vi "UseOuterEnvelope.vi"(10 "Outer Envelope Label":string) -> (3 "Translator":refnum<class "AddOuterEnvelope.lvclass">)   [LabVIEW 2011, in "Messenging.lvlib" / "AddOuterEnvelope.lvclass"]
uses:
  AddOuterEnvelope.lvclass
  AddOuterEnvelope.lvclass/AddOuterEnvelope.ctl
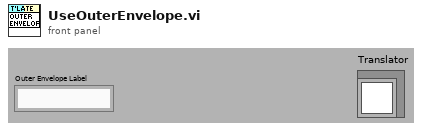
[diagram p1: front panel]
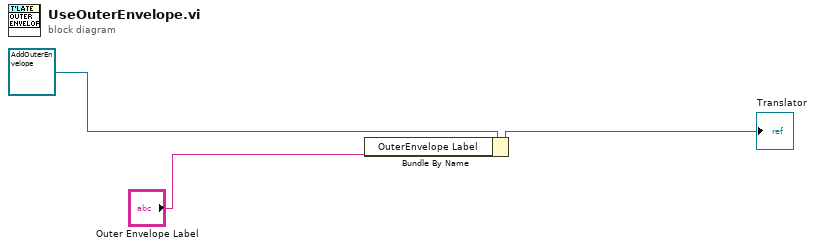
[diagram p0: block diagram]
diagram:
  n1 = Bundle By Name(cluster=refnum<class "AddOuterEnvelope.lvclass"> refnum ("SubstututeMessage in"), "OuterEnvelope Label"="Outer Envelope Label") -> (→"Translator":refnum<class "AddOuterEnvelope.lvclass">)
